vi "CAN frame Generator for Test.vi"() -> ()   [LabVIEW 2025]
uses:
  <resource>/objmgr/xnet.rc
  <vilib>/xnet/xnet.llb/XNET Create Session (Frame Output Stream).vi
  <vilib>/xnet/xnet.llb/XNET Write (Frame CAN).vi
  <vilib>/xnet/xnet.llb/XNET Frame Type CAN.ctl
  <vilib>/xnet/xnet.llb/XNET Frame CAN.ctl
panel:
  in  "Echo Transmit":bool
  in  "CAN frames":T1[](array[typedef]) {"payload" format="%x"; "timestamp" format="%<%.7X\n%x>T"; "type" items=["CAN Data"=0, "CAN Remote"=1, "CAN Bus Error"=2, "CAN 2.0 Data"=8, "CAN FD Data"=16, "CAN FD+BRS Data"=24, "J1939 Data"=192, "Delay"=224, "Log Trigger"=225, "Start Trigger"=226]; "identifier" format="%x"}
  in  "Wait time (ms)":u32=1000
  in  "Baud Rate (bps)":u64=19200
  in  "Termination":bool
  in  "CAN interface":refnum<k21>="LIN2"
  out "Instruction 2":string="Sends LIN messages to the selected interface with the selected rate (defualt is 1000 ms).\nSet \"Is Master Node\" to true when no other master node active on the bus.\n"
  in  "Stop Button 2":bool
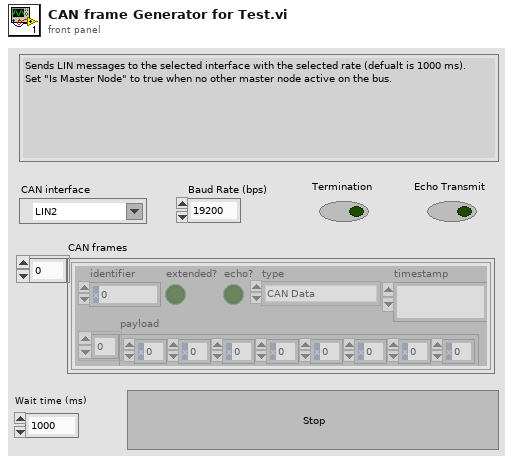
[diagram p1: front panel]
types:
  T1 = typedef "XNET Frame CAN.ctl" = cluster{"timestamp":timestamp, "payload":u8[], "identifier":u32, "type":T2, "extended?":bool, "echo?":bool}
  T2 = typedef "XNET Frame Type CAN.ctl" = u8
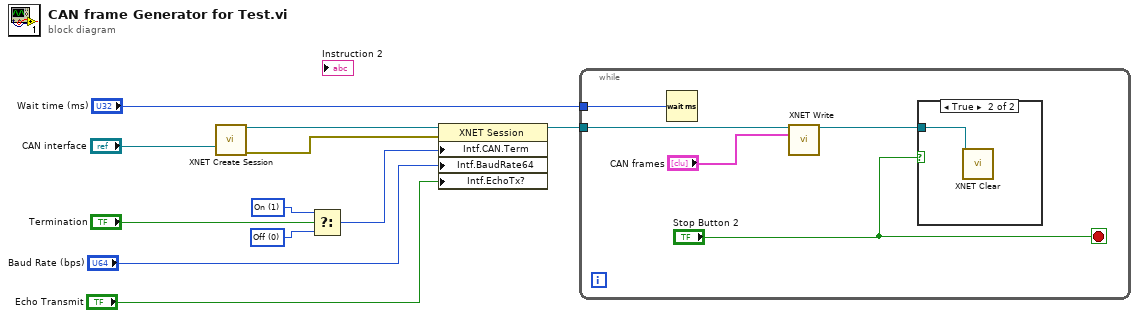
[diagram p0: block diagram]
diagram:
  w10 = u32 1 items=["Off", "On"] ("Interface:CAN:Termination")
  w11 = u32 0 items=["Off", "On"] ("Interface:CAN:Termination")
  n1 = call-poly <vilib>:"XNET Create Session.vi"("interface"="CAN interface") -> ("session out"=w7:refnum<k21>, "error out"=w8:errorcluster)  [unwired: 13 in]
  n2 = Select(t=w10, s="Termination", f=w11) -> (s? t:f=w9:u32)
  n3 = property class="XNET Session"(reference=w7, error in=w8, "Intf.CAN.Term"=w9, "Intf.BaudRate64"="Baud Rate (bps)", "Intf.EchoTx?"="Echo Transmit") -> (reference out=w3:refnum<k21>)  [unwired: 1 out]
  n4 = while {
    tunnel: w3 -> [w16]
    tunnel: "Wait time (ms)" -> [w13]
    stop <- "Stop Button 2" stop-if-true
    n5 = Wait (ms)(milliseconds to wait=w13) -> ()  [unwired: 1 out]
    n6 = call-poly <vilib>:"XNET Write.vi"("session in"=w16, "data"="CAN frames") -> ("session out"=w14:refnum<k21>)  [unwired: 12 in, 1 out]
    n7 = case shown="True" "Stop Button 2" {
      tunnel: w14 -> [_ w17]
      frame False {
      }
      frame True {
        n8 = call <vilib>:"XNET Clear.vi"("session in"=w17) -> ()  [unwired: 14 in, 1 out]
      }
    }
  }
